vi "class_data.vi"() -> ()   [LabVIEW 2010, in "SignalWriterMM140725DAQmx.lvclass"]
uses:
  SignalWriterMM140725DAQmx.lvclass
panel:
  in  "counter tasks":refnum<k21>[](array[refnum])
  out "written to devices?":bool[](array[boolean])
  in  "output tasks":refnum<k21>[](array[refnum])
  # "ATTENTION: \nEach WriteSignals plug-in possesses a single analog output (AO) channel. \nWe want it to be possible that the AO channels of multiple plug-in instances can both be distributed over different devices or reside on the same device. However, for most device types, data for channels on the same device can only be written to this device en bloc. For that reason, if a single plug-in instance writes its data to its device, it has to be aware of other instances making use of the same device and write their data as well. Via the global variables below, each plug-in instance has access to the data of other instances."
  # "- each tasks can comprise multiple channels on the same device\n- different devices are represented by different tasks"
  # "- each device has its own (and unique) entry in the array, containing the data for the corresponding task"
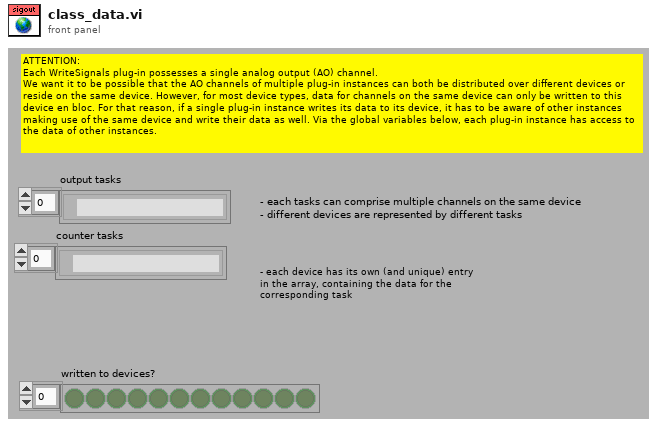
[diagram p1: front panel]
diagram:
